vi "Load and Validate.vi"(8 "error in (no error)":errorcluster, 9 "Build Config Override":path, 10 "Report Folder":path, 11 "Project Path":path) -> (0 "error out":errorcluster, 1 "Valid?":bool, 2 "Invalid Sections":string[](array[string]), 3 "Run cluster":T1)   [LabVIEW 2019, in "ProjectBuilder.lvlib" / "Project Builder.lvclass"]
doc: "Load the build config file and populate the 'Run cluster'. The loaded actions will be populated and validated."
uses:
  Project Builder.lvclass
  Ctl/Ctl_Run Cluster.ctl
  Project Action/Project Action.lvclass
  Report Action/Report Action/Report Action.lvclass
  Ctl/Ctl_Build Steps.ctl
  Project Action/Project Action.lvclass/Project Action.ctl
  PPL/HDH.ClassLoader.lvlibp
  <vilib>/Utility/config.llb/NI_LVConfig.lvlib
  ProjectBuilder.lvlib
  <vilib>/Utility/Data Type/NI_Data Type.lvlib
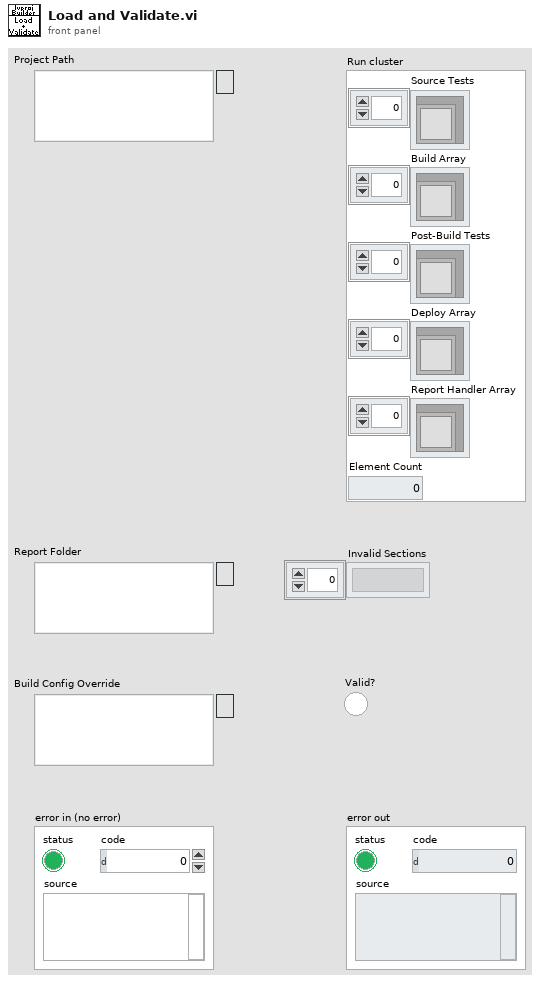
[diagram p1: front panel]
types:
  T1 = typedef "ProjectBuilder.lvlib/Project Builder.lvclass/Ctl_Run Cluster.ctl" = cluster{"Source Tests":refnum<class "Project Action.lvclass">[], "Build Array":refnum<class "Project Action.lvclass">[], "Post-Build Tests":refnum<class "Project Action.lvclass">[], "Deploy Array":refnum<class "Project Action.lvclass">[], "Report Handler Array":refnum<class "Report Action.lvclass">[], "Element Count":i32}
  T2 = typedef "ProjectBuilder.lvlib/Ctl_Build Steps.ctl" = enum16{"Source Test", "Build", "Post-Build Test", "Deploy", "Report"}
  T3 = typedef "NI_LVConfig.lvlib/Config Data RefNum.ctl" = refnum<k1>
  T4 = cluster{"Build Step":T2, "Number Array":i32[], "String":string}
  T5 = cluster{"Build Step":T2, "Number Array":i32[], "String":string}[]
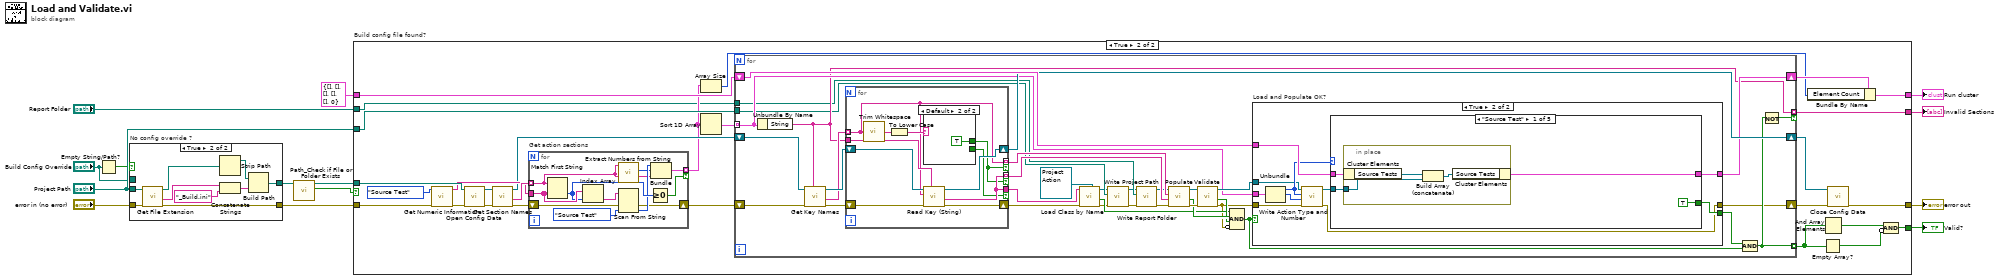
[diagram p0: block diagram]
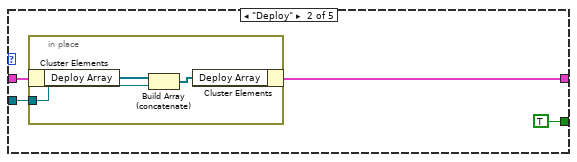
[diagram p5: hidden frame]
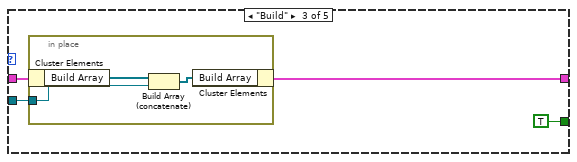
[diagram p6: hidden frame]
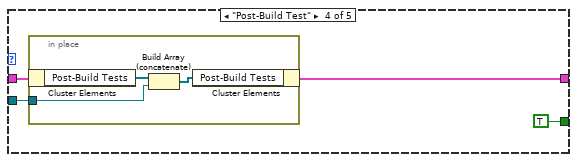
[diagram p7: hidden frame]
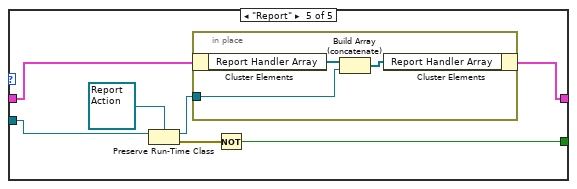
[diagram p8: hidden frame]
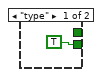
[diagram p9: hidden frame]
diagram:
  n1 = Empty String/Path?(string/path="Build Config Override") -> (empty?=w3:bool)
  n2 = case "No config override ?" shown="True" w3 {
    tunnel: "error in (no error)" -> [w16 w23]
    tunnel: [w15 w19] -> w2
    tunnel: [w16 w18] -> w11
    tunnel: "Project Path" -> [_ w17]
    tunnel: "Build Config Override" -> [w15 _]
    frame False {
    }
    frame True {
      n3 = call <vilib>:"Get File Extension.vi"("error in (no error)"=w23, "file"=w17) -> ("error out"=w18:errorcluster, "filename without extension"=w25:string, "dup file"=w22:path)  [unwired: 5 in, 2 out]
      n4 = Strip Path(path=w22) -> (stripped path=w21:path)  [unwired: 1 out]
      n5 = Concatenate Strings(w25, "_Build.ini" ("string")) -> (w20:string)
      n6 = Build Path(base path=w21, name or relative path=w20) -> (appended path=w19:path)
    }
  }
  n7 = call "Path_Check if File or Folder Exists.vi"("File or Folder Path in"=w2) -> ("File or Folder Found?"=w13:bool, "File or Folder Path dub"=w12:path)  [unwired: 9 in]
  n8 = case "Build config file found?" shown="True" w13 {
    tunnel: w12 -> [_ w54]
    tunnel: w11 -> [w27 w48]
    tunnel: [w27 w45] -> w10
    tunnel: [w26 w33] -> w9
    tunnel: T1 {"Source Tests"=[], "Build Array"=[], "Post-Build Tests"=[], "Deploy Array"=[], "Report Handler Array"=[], "Element Count"=0} ("Run Cluster") -> [w26 w38]
    tunnel: [_ w29] -> w8
    tunnel: [_ w36] -> w7
    tunnel: "Project Path" -> [_ w35]
    tunnel: "Report Folder" -> [_ w31]
    frame False {
    }
    frame True {
      n9 = call <vilib>:"Get Numeric Information.vi"("error in (no error)"=w48, "variant"=Ctl_Build_Steps."Source Test" ("Build Step")) -> ("error out"=w47:errorcluster, "enum names"=w49:string[])  [unwired: 6 in, 2 out]
      n10 = call <vilib>:"Open Config Data.vi"("error in (no error)"=w47, "configuration file path"=w54) -> ("error out"=w52:errorcluster, "refnum"=w53:T3)  [unwired: 7 in, 1 out]
      n11 = call <vilib>:"Get Section Names.vi"("error in (no error)"=w52, "refnum"=w53) -> ("error out"=w46:errorcluster, "section names"=w51:string[], "refnum out"=w41:T3)  [unwired: 7 in]
      n12 = for "Get action sections" {
        tunnel: w51 -> [w154] mode=indexing
        tunnel: w49 -> [w163]
        shift-right: [w155] -> w43
        shift-left: w46 -> [w161]
        tunnel: [w160] -> w34 mode=indexing if=w159
        n13 = Match First String(2:w163, 3:w154) -> (0:w162:i32)  [unwired: 1 out]
        n14 = Index Array(array=w163, index=w162) -> (element=w158:string)
        n15 = call "Extract Numbers from String.vi"("String"=w154) -> ("Number Array"=w153:i32[])  [unwired: 9 in, 1 out]
        n16 = Scan From String(input string=w158, error in=w161, default 1=Ctl_Build_Steps."Source Test" ("Build Step")) -> (error out=w155:errorcluster, output 1=w156:T2)  [unwired: 2 in, 2 out]
        n17 = Greater Or Equal To 0?(x=w162) -> (x >= 0?=w159:bool)
        n18 = Bundle("Build Step"=w156, "Number Array"=w153, "String"=w154) -> (w160:T4)  [unwired: 1 in]
      }
      n19 = Array Size(array=w34) -> (size(s)=w32:i32)
      n20 = Sort 1D Array(array=w34) -> (sorted array=w44:T5)
      n21 = for {
        tunnel: w44 -> [w64] mode=indexing
        shift-right: [w65] -> w42
        shift-left: w43 -> [w87]
        shift-right: [w85] -> w40
        shift-left: w41 -> [w88]
        shift-right: [w72] -> w39
        shift-left: w38 -> [w89]
        tunnel: [w70] -> w30 mode=indexing
        tunnel: [w63] -> w36 mode=indexing if=w73
        tunnel: w35 -> [w62]
        tunnel: w31 -> [w61]
        n22 = Unbundle By Name(w64) -> ("String"=w63:string)
        n23 = call <vilib>:"Get Key Names.vi"("section"=w63, "error in (no error)"=w87, "refnum"=w88) -> ("error out"=w84:errorcluster, "key names"=w83:string[], "refnum out"=w86:T3)  [unwired: 5 in, 1 out]
        n24 = for {
          shift-right: [w149] -> w85
          shift-left: w86 -> [w150]
          shift-right: [w147] -> w81
          shift-left: w84 -> [w148]
          tunnel: w83 -> [w140] mode=indexing
          tunnel: w63 -> [w146]
          tunnel: [w145] -> w78 mode=indexing if=w142
          tunnel: [w140] -> w79 mode=indexing if=w142
          tunnel: [w145] -> w82 if=w141
          n25 = call <vilib>:"Trim Whitespace.vi"("string"=w140) -> ("trimmed string"=w144:string)  [unwired: 1 in]
          n26 = To Lower Case(string=w144) -> (all lower case string=w143:string)
          n27 = case shown="Default" w143 {
            tunnel: [_ TRUE] -> w142
            tunnel: [TRUE _] -> w141
            frame "type" {
            }
            frame Default {
            }
          }
          n28 = call <vilib>:"Read Key (String).vi"("section"=w146, "error in (no error)"=w148, "key"=w140, "refnum"=w150) -> ("error out"=w147:errorcluster, "value"=w145:string, "refnum out"=w149:T3)  [unwired: 4 in, 1 out]
        }
        n29 = call "Load Class by Name.vi"("Class Type"=refnum<class "Project Action.lvclass"> refnum ("ProjectBuilder.lvlib:Project Action.lvclass"), "error in (no error)"=w81, "Base Class Name"=w82) -> ("error out"=w57:errorcluster, "Load and Type Success?"=w68:bool, "Loaded Class"=w60:refnum<class "Project Action.lvclass">)  [unwired: 5 in, 1 out]
        n30 = call "Write Project Path.vi"("error in (no error)"=w57, "Project Path"=w62, "Project Action in"=w60) -> ("error out"=w56:errorcluster, "Project Action out"=w59:refnum<class "Project Action.lvclass">)  [unwired: 7 in]
        n31 = call "Write Report Folder.vi"("error in (no error)"=w56, "Report Folder"=w61, "Project Action in"=w59) -> ("error out"=w55:errorcluster, "Project Action out"=w58:refnum<class "Project Action.lvclass">)  [unwired: 7 in]
        n32 = call "Populate.vi"("error in (no error)"=w55, "Values"=w78, "Names"=w79, "Action Interface in"=w58) -> ("error out"=w80:errorcluster, "Success?"=w77:bool, "Action Interface out"=w76:refnum<class "Project Action.lvclass">)  [unwired: 5 in]
        n33 = call "Validate.vi"("error in (no error)"=w80, "Action Interface in"=w76) -> ("error out"=w66:errorcluster, "Valid?"=w74:bool, "Action Interface out"=w75:refnum<class "Project Action.lvclass">)  [unwired: 7 in]
        n34 = Compound Arithmetic op=AND(w68, w77, w74, invert w66) -> (w71:bool)
        n35 = case "Load and Populate OK?" shown="True" w71 {
          tunnel: w89 -> [w91 w101]
          tunnel: w75 -> [_ w93]
          tunnel: [w91 w100] -> w72
          tunnel: [_ w99] -> w67
          tunnel: [w90 w98] -> w65
          tunnel: w66 -> [w90 w92]
          tunnel: w64 -> [_ w96]
          frame False {
          }
          frame True {
            n36 = Unbundle(w96) -> ("Build Step"=w95:T2, "Number Array"=w94:i32[])  [unwired: 1 out]
            n37 = call "Write Action Type and Number.vi"("error in (no error)"=w92, "Action Number"=w94, "Action Type"=w95, "Project Action in"=w93) -> ("error out"=w98:errorcluster, "Project Action out"=w97:refnum<class "Project Action.lvclass">)  [unwired: 6 in]
            n38 = case shown="\"Source Test\"" w95 {
              tunnel: w101 -> [w104 w112 w118 w125 w134]
              tunnel: w97 -> [w105 w110 w119 w126 w136]
              tunnel: [w103 w111 w117 w124 w132] -> w100
              tunnel: [TRUE TRUE TRUE TRUE w130] -> w99
              frame "Source Test" {
                n39 = in-place {
                  in-place-border: w105 -> [w107]
                  n40 = in-place-cluster #1(w104) -> ("Source Tests"=w108:refnum<class "Project Action.lvclass">[])
                  n41 = Build Array (concatenate)(w108, w107) -> (w106:refnum<class "Project Action.lvclass">[])
                  n42 = in-place-cluster #1("Source Tests"=w106) -> (w103:T1)
                }
              }
              frame "Deploy" {
                n43 = in-place {
                  in-place-border: w110 -> [w114]
                  n44 = in-place-cluster #2(w112) -> ("Deploy Array"=w115:refnum<class "Project Action.lvclass">[])
                  n45 = Build Array (concatenate)(w115, w114) -> (w113:refnum<class "Project Action.lvclass">[])
                  n46 = in-place-cluster #2("Deploy Array"=w113) -> (w111:T1)
                }
              }
              frame "Build" {
                n47 = in-place {
                  in-place-border: w119 -> [w121]
                  n48 = in-place-cluster #3(w118) -> ("Build Array"=w122:refnum<class "Project Action.lvclass">[])
                  n49 = Build Array (concatenate)(w122, w121) -> (w120:refnum<class "Project Action.lvclass">[])
                  n50 = in-place-cluster #3("Build Array"=w120) -> (w117:T1)
                }
              }
              frame "Post-Build Test" {
                n51 = in-place {
                  in-place-border: w126 -> [w128]
                  n52 = in-place-cluster #4(w125) -> ("Post-Build Tests"=w129:refnum<class "Project Action.lvclass">[])
                  n53 = Build Array (concatenate)(w129, w128) -> (w127:refnum<class "Project Action.lvclass">[])
                  n54 = in-place-cluster #4("Post-Build Tests"=w127) -> (w124:T1)
                }
              }
              frame "Report" {
                n55 = Preserve Run-Time Class(object in=w136, 2:refnum<class "Report Action.lvclass"> refnum ("ProjectBuilder.lvlib:Report Handler.lvclass")) -> (object out=w133:refnum<class "Report Action.lvclass">, error out=w131:errorcluster)  [unwired: 1 in]
                n56 = in-place {
                  in-place-border: w133 -> [w138]
                  n57 = in-place-cluster #5(w134) -> ("Report Handler Array"=w139:refnum<class "Report Action.lvclass">[])
                  n58 = Build Array (concatenate)(w139, w138) -> (w137:refnum<class "Report Action.lvclass">[])
                  n59 = in-place-cluster #5("Report Handler Array"=w137) -> (w132:T1)
                }
                n60 = Not(x=w131) -> (.not. x?=w130:bool)
              }
            }
          }
        }
        n61 = Compound Arithmetic op=AND(w67, w71) -> (w70:bool)
        n62 = Not(x=w70) -> (.not. x?=w73:bool)
      }
      n63 = Bundle By Name(cluster=w39, "Element Count"=w32) -> (w33:T1)
      n64 = And Array Elements(Boolean array=w30) -> (logical AND=w37:bool)
      n65 = Empty Array?(array=w30) -> (empty?=w28:bool)
      n66 = call <vilib>:"Close Config Data.vi"("error in (no error)"=w42, "refnum"=w40) -> ("error out"=w45:errorcluster)  [unwired: 8 in, 1 out]
      n67 = Compound Arithmetic op=AND(w37, invert w28) -> (w29:bool)
    }
  }
  "error out" <- w10
  "Run cluster" <- w9
  "Valid?" <- w8
  "Invalid Sections" <- w7
